vi "Write Signal Generator (0=none).vi"(10 "Signal Generator (0=none)":i32, 11 "Switching Time in":refnum<class "Switching Time.lvclass">) -> (3 "Switching Time out":refnum<class "Switching Time.lvclass">)   [LabVIEW 2020, in "Switching Time.lvclass"]
uses:
  Switching Time.lvclass
  Switching Time.lvclass/Switching Time.ctl
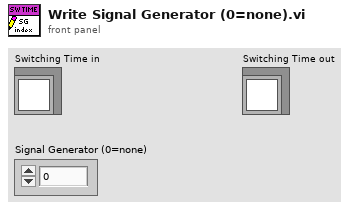
[diagram p1: front panel]
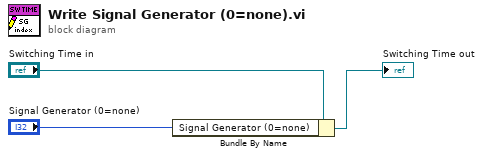
[diagram p0: block diagram]
diagram:
  n1 = Bundle By Name(cluster="Switching Time in", "Signal Generator (0=none)"="Signal Generator (0=none)") -> (→"Switching Time out":refnum<class "Switching Time.lvclass">)
